vi "String - Split Array of Command and Access Control Strings.vi"(11 "Commands and RW Properties":string[](array[string])) -> (1 "Write Access":bool[](array[boolean]), 2 "Read Access":bool[](array[boolean]), 3 "Commands":string[](array[string]))   [LabVIEW 2017, in "Communications Library.lvlib"]
doc: "Deciphers an array of strings from the response to the help2 command."
uses:
  Communications Library.lvlib
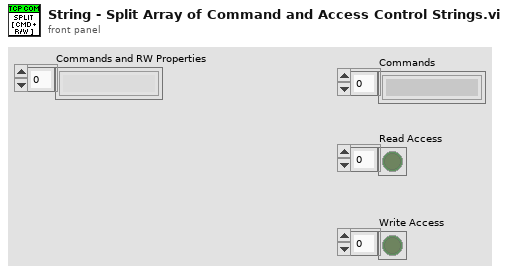
[diagram p1: front panel]
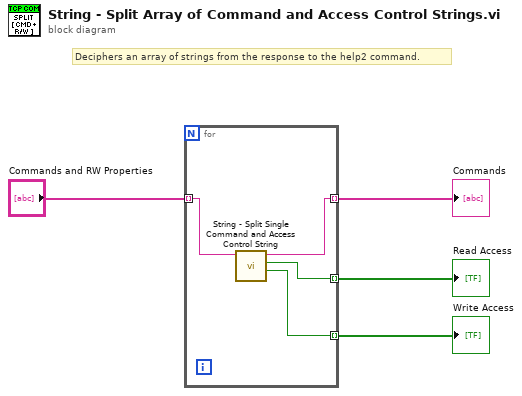
[diagram p0: block diagram]
diagram:
  # "Deciphers an array of strings from the response to the help2 command."
  n1 = for {
    tunnel: "Commands and RW Properties" -> [w8] mode=indexing
    tunnel: [w7] -> w4 mode=indexing
    tunnel: [w6] -> w2 mode=indexing
    tunnel: [w5] -> w1 mode=indexing
    n2 = call "String - Split Single Command and Access Control String.vi"("Command and RW Property"=w8) -> ("Write Access"=w5:bool, "Read Access"=w6:bool, "Command"=w7:string)  [unwired: 8 in]
  }
  "Commands" <- w4
  "Read Access" <- w2
  "Write Access" <- w1
